vi "PythonName.vi"(6 "add self":bool, 8 "error in":errorcluster, 11 "Terminal in":refnum<class "Terminal.lvclass">) -> (0 "error out":errorcluster, 3 "Terminal out":refnum<class "Terminal.lvclass">, 5 "name":string, 7 "UID":string)   [LabVIEW 2014, in "Terminal.lvclass"]
uses:
  Terminal.lvclass
  Python/Parsing/Python Functions.lvlib
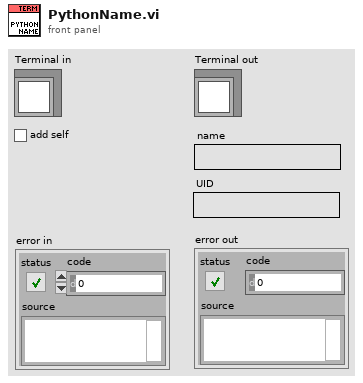
[diagram p1: front panel]
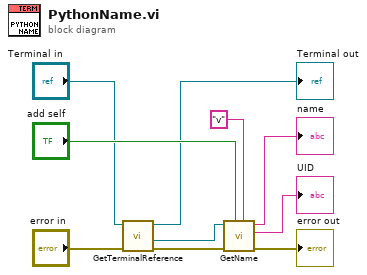
[diagram p0: block diagram]
diagram:
  n1 = call "GetTerminalReference.vi"("error in"="error in", "Terminal in"="Terminal in") -> ("error out"=w5:errorcluster, "reference"=w4:refnum<vi>, "Terminal out"=→"Terminal out":refnum<class "Terminal.lvclass">)  [unwired: 7 in]
  n2 = call "GetName.vi"("base name"="v", "add self"="add self", "error in"=w5, "GObj Refnum"=w4) -> ("error out"=→"error out":errorcluster, "UID"=→"UID":string, "name"=→"name":string)  [unwired: 5 in]
